vi "Init.vi"(8 "error in (no error)":errorcluster, 11 "Data in":refnum<class "Polled_EventSource.lvclass">) -> (0 "error out":errorcluster, 3 "Data out":refnum<class "Polled_EventSource.lvclass">)   [LabVIEW 2021, in "Polled_EventSource.lvclass"]
doc: "Abstract Data Classes 2.1.1.13\nTim Streeter - TSA\nCopyright (c) 2025, TSA"
uses:
  Polled_EventSource.lvclass
  Polled_EventSource.lvclass/Polled_EventSource.ctl
  Support/Actor.vi
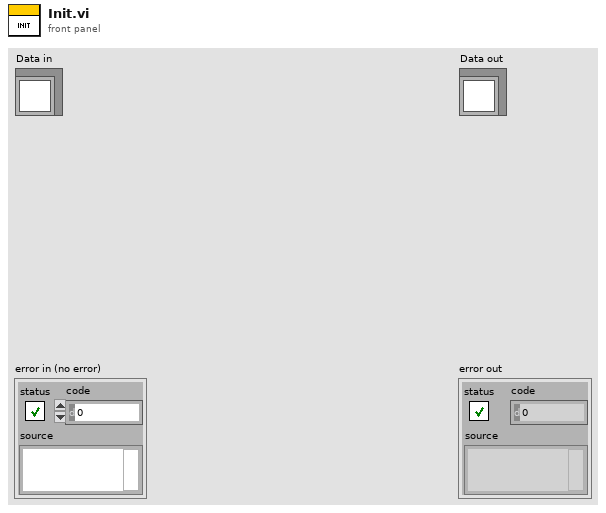
[diagram p1: front panel]
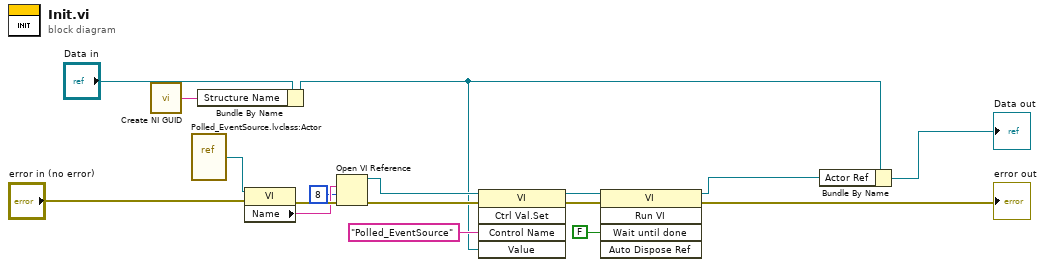
[diagram p0: block diagram]
diagram:
  n1 = call <vilib>:"Create NI GUID.vi"() -> ("NI GUID"=w5:string)
  n2 = vi-ref "Polled_EventSource.lvclass:Actor.vi"() -> (w17:refnum<vi>)
  n3 = Bundle By Name(cluster="Data in", "Structure Name"=w5) -> (w4:refnum<class "Polled_EventSource.lvclass">)
  n4 = property class="VI"(reference=w17, error in="error in (no error)") -> (error out=w15:errorcluster, "Name"=w14:string)  [unwired: 1 out]
  n5 = Open VI Reference(vi path=w14, options=8, error in (no error)=w15) -> (vi reference=w7:refnum<vi>, error out=w8:errorcluster)  [unwired: 3 in]
  n6 = invoke class="VI" method="Ctrl Val.Set"(reference=w7, error in=w8, "Control Name"="Polled_EventSource", "Value"=w4) -> (reference out=w9:refnum<vi>, error out=w10:errorcluster)  [unwired: 1 in, 3 out]
  n7 = invoke class="VI" method="Run VI"(reference=w9, error in=w10, "Wait until done"=FALSE ("Wait Until Done")) -> (reference out=w1:refnum<vi>, error out=→"error out":errorcluster)  [unwired: 2 in, 3 out]
  n8 = Bundle By Name(cluster=w4, "Actor Ref"=w1) -> (→"Data out":refnum<class "Polled_EventSource.lvclass">)
